vi "Find Value.vi"(0 "Key":string, 1 "Data":cluster{"Key":string, "Value":variant}[](array[cluster])) -> (2 "Value":variant, 3 "Found?":bool)   [LabVIEW 2018, in "Toolkit.lvlib" / "Nodes.lvlib" / "NonTerminal.lvclass"]
uses:
  NonTerminal.lvclass
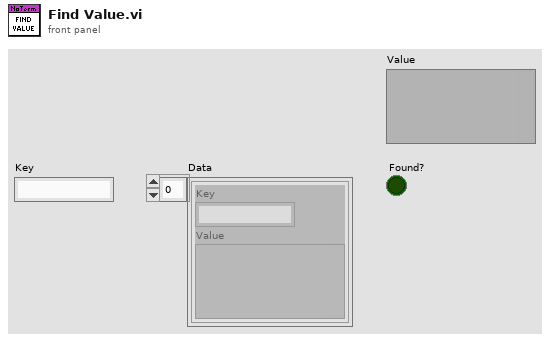
[diagram p1: front panel]
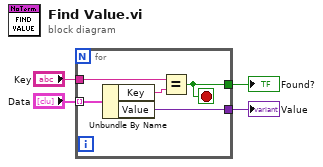
[diagram p0: block diagram]
diagram:
  n1 = for {
    tunnel: "Data" -> [w9] mode=indexing
    tunnel: "Key" -> [w7]
    tunnel: [w6] -> w1
    tunnel: [w5] -> w2
    stop <- w6 stop-if-true
    n2 = Unbundle By Name(w9) -> ("Key"=w8:string, "Value"=w5:variant)
    n3 = Equal?(x=w7, y=w8) -> (x = y?=w6:bool)
  }
  "Value" <- w2
  "Found?" <- w1
